vi "IPC-Modbus-Transfer-GetMBAP.vi"(8 "错误输入（无错误）":errorcluster, 11 "connection ID in":refnum<k5>) -> (0 "错误输出":errorcluster, 2 "MBAP":T1, 3 "连接ID输出":refnum<k5>)   [LabVIEW 2014]
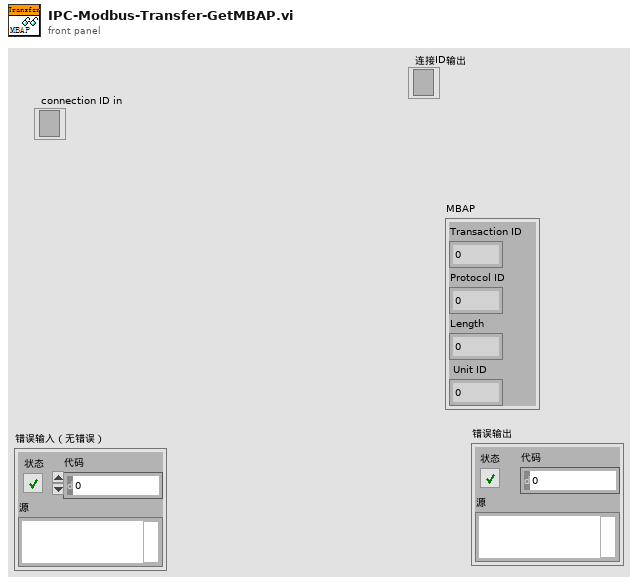
[diagram p1: front panel]
types:
  T1 = cluster{"Transaction ID":u16, "Protocol ID":u16, "Length":u16, " Unit ID":u8}
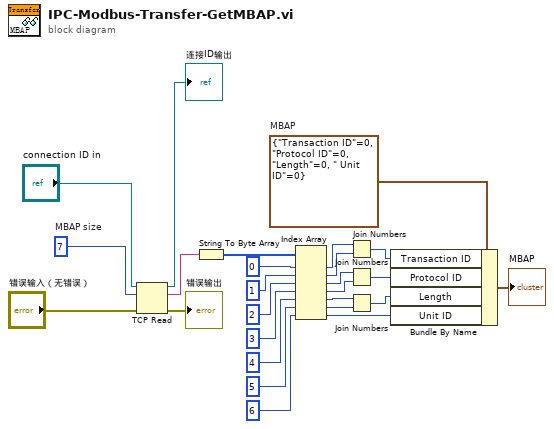
[diagram p0: block diagram]
diagram:
  w12 = T1 {"Transaction ID"=0, "Protocol ID"=0, "Length"=0, " Unit ID"=0}  # MBAP
  w26 = 7  # MBAP size
  n1 = TCP Read(connection ID="connection ID in", bytes to read=w26, error in (no error)="错误输入（无错误）") -> (connection ID out=→"连接ID输出":refnum<k5>, data out=w21:string, error out=→"错误输出":errorcluster)  [unwired: 2 out]
  n2 = String To Byte Array(string=w21) -> (unsigned byte array=w20:u8[])
  n3 = Index Array(array=w20, index #1=0 ("索引"), index #2=1 ("索引"), index #3=2 ("索引"), index #4=3 ("索引"), index #5=4 ("索引"), index #6=5 ("索引"), index #7=6 ("索引")) -> (element #1=w11:u8, element #2=w10:u8, element #3=w8:u8, element #4=w7:u8, element #5=w5:u8, element #6=w4:u8, element #7=w2:u8)
  n4 = Join Numbers(hi=w11, lo=w10) -> ((hi.lo)=w9:u16)
  n5 = Join Numbers(hi=w8, lo=w7) -> ((hi.lo)=w6:u16)
  n6 = Join Numbers(hi=w5, lo=w4) -> ((hi.lo)=w3:u16)
  n7 = Bundle By Name(cluster=w12, "Transaction ID"=w9, "Protocol ID"=w6, "Length"=w3, "Unit ID"=w2) -> (→"MBAP":T1)
